vi "Finish.vi"   [LabVIEW 2016]
doc: "This VI is called during exit. It can be used to close I/O refnums, save collected data, etc."
uses:
  <vilib>/Rock Robotics/WPI/Utilities/WPI_GetSetVariantRefNum.vi
types:
  T1 = typedef "WPI_I2CDevRef.ctl" = cluster{"DevStatus":errorcluster, "Device Address":u8, "Handle":i32, "I2C Bus":T2}
  T2 = typedef "i2c_bus.ctl" = enum16{"I2C On-Board", "I2C MXP", "Invalid"}
  T3 = typedef "WPI_JoystickDevRef.ctl" = cluster{"Device":T4}
  T4 = typedef "WPI_JoystickDeviceEnum.ctl" = enum16{"USB 0", "USB 1", "USB 2", "USB 3", "USB 4", "USB 5"}
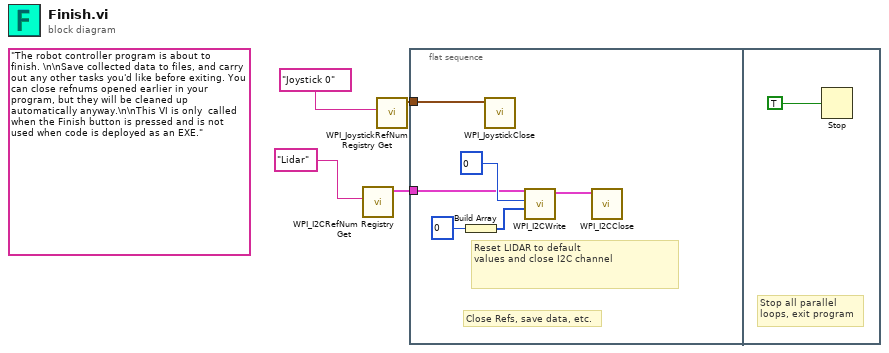
[diagram p0: block diagram]
diagram:
  (unwired) "The robot controller program is about to finish. \n\nSave collected data to files, and carry out any other tasks you'd like before exiting. You can close refnums opened earlier in your program, but they will be cleaned up automatically anyway.\n\nThis VI is only  called when the Finish button is pressed and is not used when code is deployed as an EXE."
  n1 = call <vilib>:"WPI_I2CRefNum Registry Get.vi"("refnum name"="Lidar") -> ("I2CDevRef"=w1:T1)  [unwired: 9 in, 1 out]
  n2 = call <vilib>:"WPI_JoystickRefNum Registry Get.vi"("refnum name"="Joystick 0") -> ("JoystickDevRef"=w3:T3)  [unwired: 1 in, 9 out]
  n3 = flat-sequence {
    tunnel: w3 -> [w10]
    tunnel: w1 -> [w5]
    frame #0 {
      # "Reset LIDAR to default\nvalues and close I2C channel"
      # "Close Refs, save data, etc."
      n4 = Build Array(u8 0 ("Device Address")) -> (w7:u8[])
      n5 = call <vilib>:"WPI_JoystickClose.vi"("JoystickDevRef"=w10) -> ()  [unwired: 11 out]
      n6 = call <vilib>:"WPI_I2CWrite.vi"("I2CDataToSend"=w7, "I2CRegister"=u8 0 ("Device Address"), "I2CDevRef"=w5) -> ("I2CDevRef"=w6:T1)  [unwired: 7 in, 1 out]
      n7 = call <vilib>:"WPI_I2CClose.vi"("I2CDevRef"=w6) -> ()  [unwired: 10 in, 1 out]
    }
    frame #1 {
      # "Stop all parallel\nloops, exit program"
      n8 = Stop(stop? (T)=TRUE ("Quit")) -> ()
    }
  }
